vi "Cleanup Default Value Template.vi"(8 "error in":errorcluster, 11 "temporary template path":path) -> (0 "error out":errorcluster)   [LabVIEW 2021, in "NI Measurement V2 Client Generator Runtime.lvlib"]
uses:
  NI Measurement V2 Client Generator Runtime.lvlib
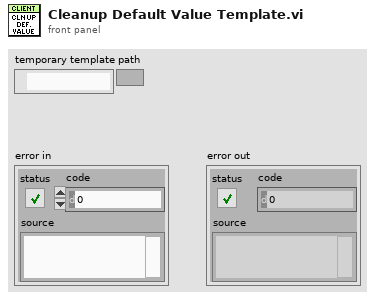
[diagram p1: front panel]
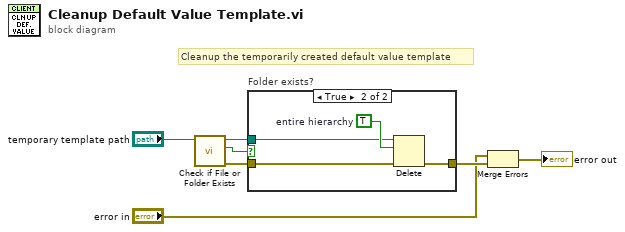
[diagram p0: block diagram]
diagram:
  # "Cleanup the temporarily created default value template"
  n1 = call <vilib>:"Check if File or Folder Exists.vi"("path"="temporary template path") -> ("error out"=w7:errorcluster, "file or folder exists?"=w6:bool, "dup path"=w5:path)  [unwired: 8 in]
  n2 = case "Folder exists?" shown="True" w6 {
    tunnel: [w8 w9] -> w3
    tunnel: w7 -> [w8 w10]
    tunnel: w5 -> [_ w11]
    frame False {
    }
    frame True {
      w12 = TRUE  # entire hierarchy
      n3 = Delete(path (use dialog)=w11, entire hierarchy (F)=w12, error in=w10) -> (error out=w9:errorcluster)  [unwired: 2 in, 2 out]
    }
  }
  n4 = Merge Errors("error in", w3) -> (→"error out":errorcluster)
